vi "copySocketReportFile.vi"   [LabVIEW 2012]
uses:
  Global1.vi
  <vilib>/Utility/file.llb/Read From Spreadsheet File (string).vi
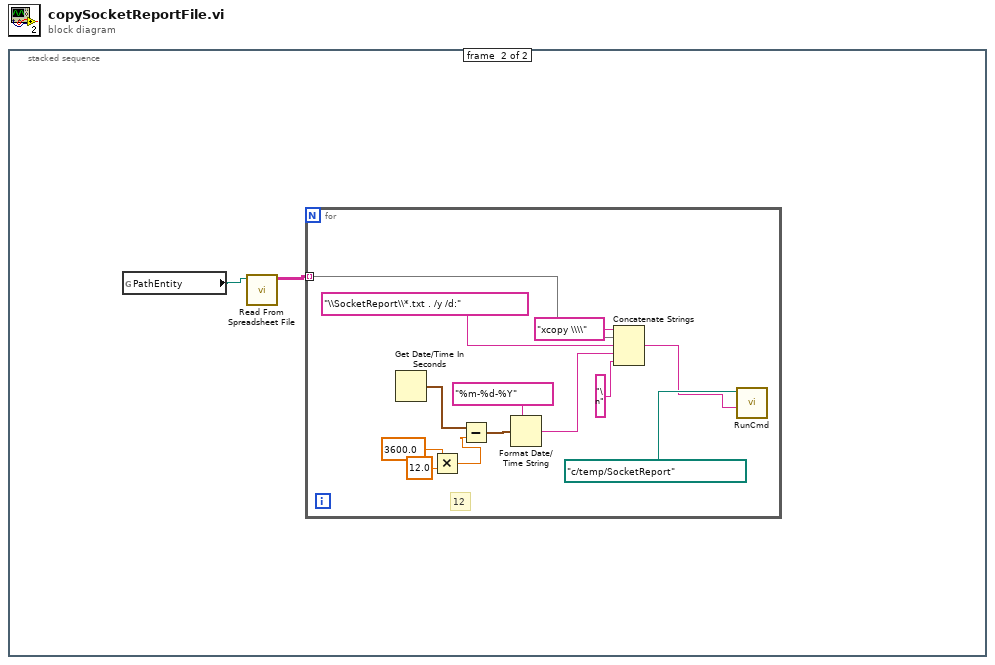
[diagram p0: block diagram]
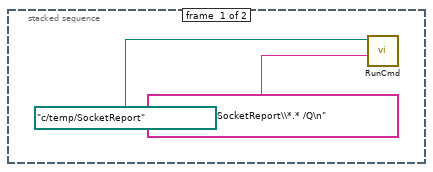
[diagram p2: hidden frame]
diagram:
  n1 = stacked-sequence {
    frame #0 {
      n2 = call "RunCmd.vi"("Cmd String"="del c:\\temp\\SocketReport\\*.* /Q\n", "working directory"=path "c:/temp/SocketReport") -> ()  [unwired: 8 in, 2 out]
    }
    frame #1 {
      n3 = global read "Global1.vi" "PathEntity"() -> (w4:path)
      n4 = call-poly <vilib>:"Read From Spreadsheet File.vi"("file path (dialog if empty)"=w4) -> ("all rows"=w3:string[][])  [unwired: 6 in, 4 out]
      n5 = for {
        tunnel: w3 -> [w8] mode=indexing
        # "12"
        n6 = Get Date/Time In Seconds() -> (seconds since 1Jan1904=w10:timestamp)
        n7 = Multiply(x=3600.0, y=12.0) -> (x*y=w12:dbl)
        n8 = Subtract(x=w10, y=w12) -> (x-y=w13:timestamp)
        n9 = Format Date/Time String(time format string (%c)="%m-%d-%Y", seconds (now)=w13) -> (date/time string=w15:string)  [unwired: 1 in]
        n10 = Concatenate Strings("xcopy \\\\" ("string"), w8, "\\SocketReport\\*.txt . /y /d:" ("string"), w15, "\n" ("string")) -> (w5:string)
        n11 = call "RunCmd.vi"("Cmd String"=w5, "working directory"=path "c:/temp/SocketReport") -> ()  [unwired: 8 in, 2 out]
      }
    }
  }
